vi "fit calibrazione.vi"(10 "data":T3, 11 "Spectrum - Background":dbl[](array[numeric])) -> (1 "intercept":dbl, 2 "slope":dbl, 3 "Ch_Ene":cluster{"Array":dbl[], "Array":dbl[]})   [LabVIEW 2023]
uses:
  <vilib>/Analysis/1siggen.llb/Ramp Pattern by Samples.vi
  <vilib>/Analysis/NI_AALBase.lvlib
  <vilib>/Analysis/NI_AALPro.lvlib
panel:
  out "index of element":i32
  out "fractional index or x":dbl
  in  "parameter bounds":T1={"amp min"=-inf, "amp max"=inf, "center min"=-inf, "center max"=inf, "deviation min"=5.0, "deviation max"=200.0, "offset min"=0.0, "offset max"=inf}
  out "XY Graph":T2(graph)
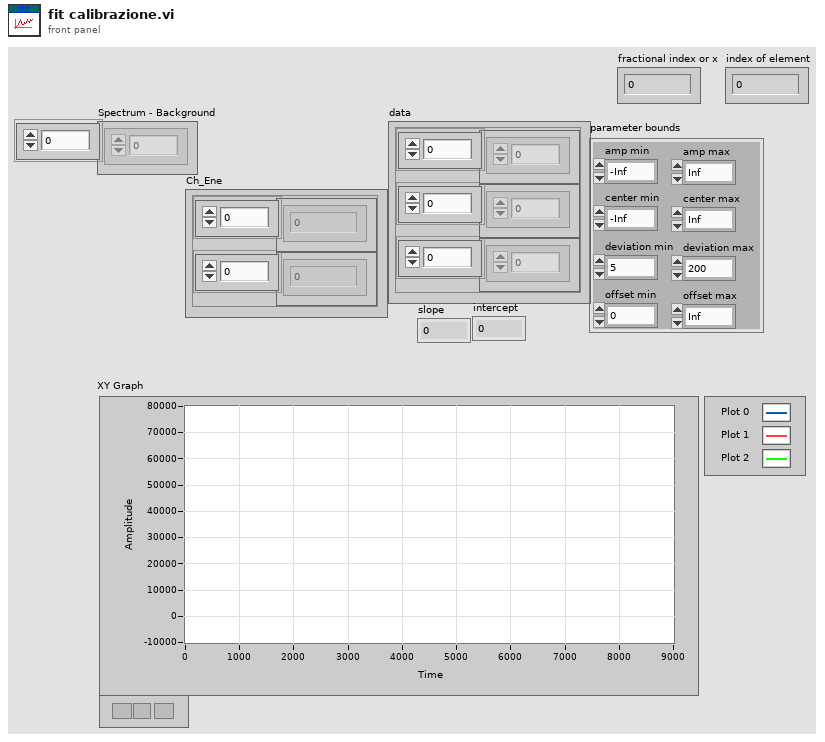
[diagram p1: front panel]
types:
  T1 = cluster{"amp min":dbl, "amp max":dbl, "center min":dbl, "center max":dbl, "deviation min":dbl, "deviation max":dbl, "offset min":dbl, "offset max":dbl}
  T2 = cluster{"Ramp Pattern":dbl[], "Spectrum - Background":dbl[]}[]
  T3 = cluster{"Array":dbl[], "Array":dbl[], "Array":dbl[]}
  T4 = cluster{"Ramp Pattern":dbl[], "Spectrum - Background":dbl[]}
  T5 = cluster{"initial amplitude":dbl, "initial center":dbl, "initial standard deviation":dbl, "offset":dbl}
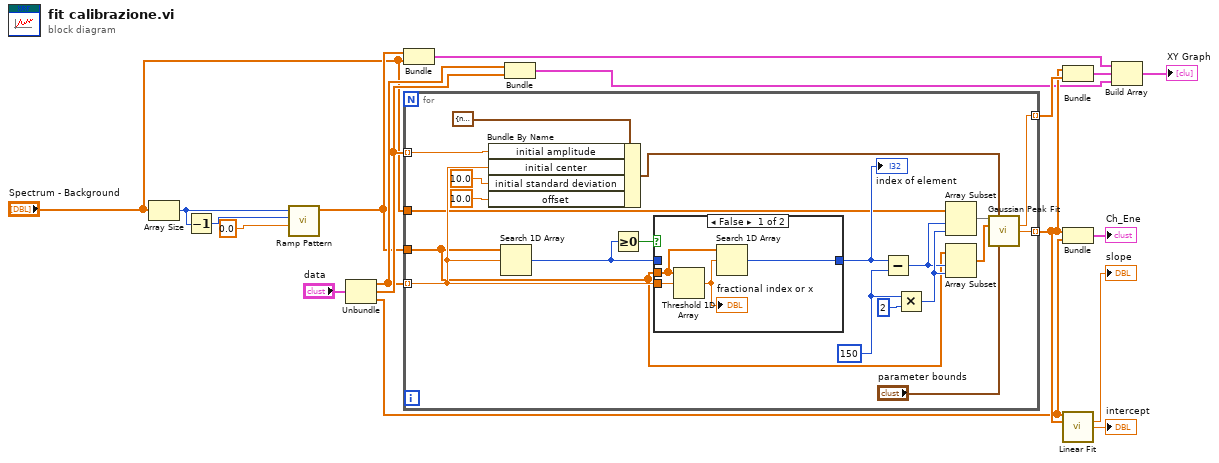
[diagram p0: block diagram]
diagram:
  n1 = Array Size(array="Spectrum - Background") -> (size(s)=w16:i32)
  n2 = Decrement(x=w16) -> (x-1=w17:i32)
  n3 = call-poly <vilib>:"Ramp Pattern.vi"("start"=0.0, "end"=w17, "samples"=w16) -> ("Ramp Pattern"=w2:dbl[])  [unwired: 7 in, 1 out]
  n4 = Unbundle("data") -> ("Array"=w3:dbl[], "Array"=w5:dbl[], "Array"=w7:dbl[])
  n5 = Bundle("Ramp Pattern"=w2, "Spectrum - Background"="Spectrum - Background") -> (w14:T4)  [unwired: 1 in]
  n6 = for {
    tunnel: w3 -> [w23] mode=indexing
    tunnel: "Spectrum - Background" -> [w22]
    tunnel: w2 -> [w21]
    tunnel: w5 -> [w37] mode=indexing
    tunnel: [w34] -> w8 mode=indexing
    tunnel: [w32] -> w9 mode=indexing
    w25 = 150 ("y")
    n7 = Bundle By Name(cluster=T5 {"initial amplitude"=nan, "initial center"=nan, "initial standard deviation"=nan, "offset"=nan} ("initial guess"), "initial amplitude"=w37, "initial center"=w23, "initial standard deviation"=10.0, "offset"=10.0) -> (w36:T5)
    n8 = Search 1D Array(1D array=w21, element=w23) -> (index of element=w27:i32)  [unwired: 1 in]
    n9 = Greater Or Equal To 0?(x=w27) -> (x >= 0?=w26:bool)
    n10 = case shown="False" w26 {
      tunnel: w21 -> [w41 _]
      tunnel: w23 -> [w42 _]
      tunnel: [w39 w43] -> w28
      tunnel: w27 -> [_ w43]
      frame False {
        n11 = Threshold 1D Array(2:w42, 3:w41) -> (0:w40:dbl)  [unwired: 1 in]
        "fractional index or x" <- w40
        n12 = Search 1D Array(1D array=w41, element=w40) -> (index of element=w39:i32)  [unwired: 1 in]
      }
      frame True {
      }
    }
    "index of element" <- w28
    n13 = Subtract(x=w28, y=w25) -> (x-y=w29:i32)
    n14 = Multiply(x=w25, y=2) -> (x*y=w30:i32)
    n15 = Array Subset(array=w22, index=w29, length=w30) -> (w20:dbl[])
    n16 = Array Subset(array=w21, index=w29, length=w30) -> (w19:dbl[])
    n17 = call <vilib>:"Gaussian Peak Fit.vi"("Y"=w20, "initial guess"=w36, "X"=w19, "parameter bounds"="parameter bounds") -> ("amplitude"=w32:dbl, "center"=w34:dbl)  [unwired: 5 in, 5 out]
  }
  n18 = Bundle("Array"=w3, "Array"=w5) -> (w4:cluster{"Array":dbl[], "Array":dbl[]})  [unwired: 1 in]
  n19 = Bundle(w8, w9) -> (w13:cluster{dbl[], dbl[]})  [unwired: 1 in]
  n20 = Bundle(w8, "Array"=w7) -> (→"Ch_Ene":cluster{dbl[], "Array":dbl[]})  [unwired: 1 in]
  n21 = call <vilib>:"Linear Fit.vi"("Y"=w7, "X"=w8) -> ("slope"=→"slope":dbl, "intercept"=→"intercept":dbl)  [unwired: 9 in, 3 out]
  n22 = Build Array(w14, w13, w4) -> (→"XY Graph":cluster{"Array":dbl[], "Array":dbl[]}[])
